vi "Read Amplitude.vi"(8 "error in (no error)":errorcluster, 11 "Analog Waveform in":refnum<class "Analog Waveform.lvclass">) -> (0 "error out":errorcluster, 2 "Amplitude":dbl, 3 "Analog Waveform out":refnum<class "Analog Waveform.lvclass">)   [LabVIEW 2020, in "Analog Waveform.lvclass"]
uses:
  Analog Waveform.lvclass
  Analog Waveform.lvclass/Analog Waveform.ctl
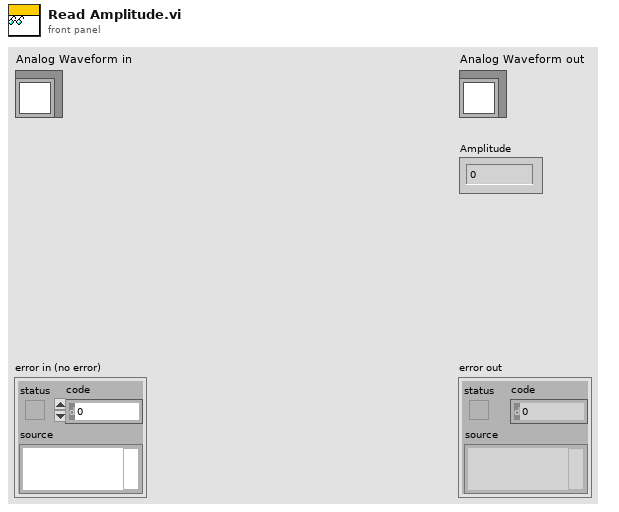
[diagram p1: front panel]
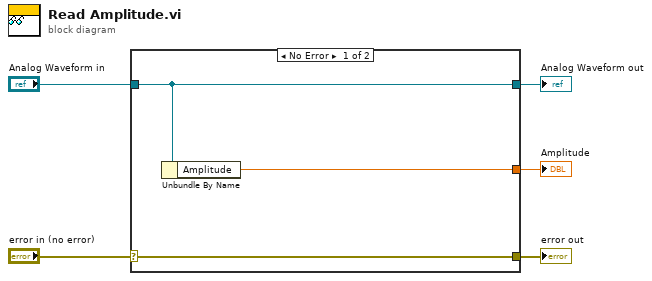
[diagram p0: block diagram]
diagram:
  n1 = case shown="No Error" "error in (no error)" {
    selector: "error in (no error)" -> [w8 w9]
    tunnel: [w8 w9] -> w4
    tunnel: [w7 w10] -> w2
    tunnel: "Analog Waveform in" -> [w7 w10]
    tunnel: [w6 _] -> w1
    frame No Error {
      n2 = Unbundle By Name(w7) -> ("Amplitude"=w6:dbl)
    }
    frame Error {
    }
  }
  "error out" <- w4
  "Analog Waveform out" <- w2
  "Amplitude" <- w1
